vi "configure.vi"(4 "error in (no error)":errorcluster, 5 "py interface file":path, 6 "Request data":variant, 7 "Python session in":refnum<k35>) -> (0 "error out":errorcluster, 2 "Response data":variant, 3 "Python session out":refnum<k35>)   [LabVIEW 2022 SP3]
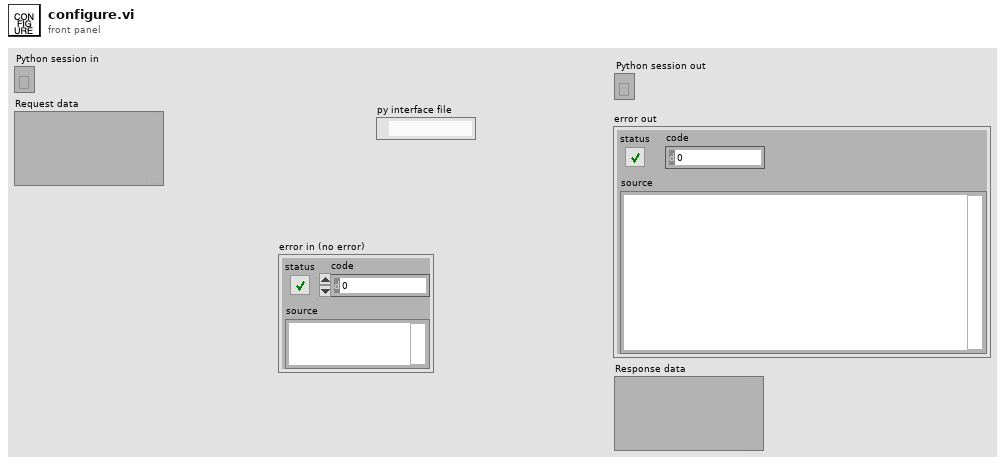
[diagram p1: front panel]
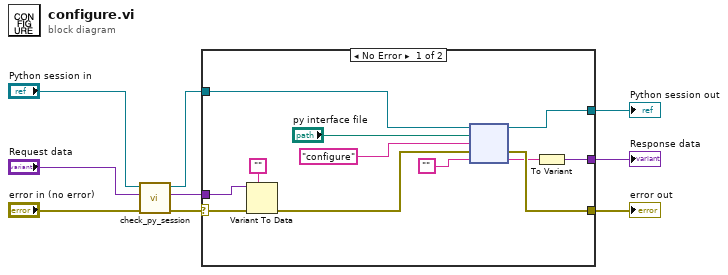
[diagram p0: block diagram]
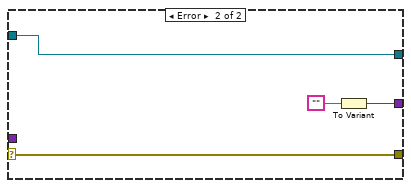
[diagram p2: hidden frame]
diagram:
  n1 = call "check_py_session.vi"("error in"="error in (no error)", "Request data"="Request data", "Python session in"="Python session in") -> ("error out"=w3:errorcluster, "Response data"=w4:variant, "Python session out"=w5:refnum<k35>)  [unwired: 2 in]
  n2 = case shown="No Error" w3 {
    selector: w3 -> [w16 w25]
    tunnel: w5 -> [w21 w24]
    tunnel: [w18 w24] -> w9
    tunnel: w4 -> [w17 _]
    tunnel: [w14 w25] -> w2
    tunnel: [w12 w22] -> w1
    frame No Error {
      n3 = Variant To Data(error in=w16, type="", Variant=w17) -> (error out=w15:errorcluster)  [unwired: 1 out]
      n4 = node(w21, "py interface file", "configure" ("function name"), w15, "") -> (w18:refnum<k35>, w14:errorcluster, w13:string)  [unwired: 2 out]
      n5 = To Variant(anything=w13) -> (Variant=w12:variant)
    }
    frame Error {
      n6 = To Variant(anything="") -> (Variant=w22:variant)
    }
  }
  "error out" <- w2
  "Python session out" <- w9
  "Response data" <- w1
